vi "ERDFind.vi"(8 "error in":errorcluster, 10 "Read ERD List":T1[](array[typedef]) {"ERD Number" format="%.0x"}, 11 "ERD Data In":cluster{"ERD Number":u16, "Data":string}[](array[cluster])) -> (0 "error out":errorcluster, 1 "Read ERD List Out":T1[](array[typedef]) {"ERD Number" format="%.0x"}, 2 "ERD Data Out":cluster{"ERD Number":u16, "Data":string}[](array[cluster]) {"ERD Number" format="%.0x"}, 3 "ERD's No Found":string[](array[string]))   [LabVIEW 2021]
uses:
  Common/LabVIEW GEA2 Toolkit/GEA3/type defs/ERD Read Data In.ctl
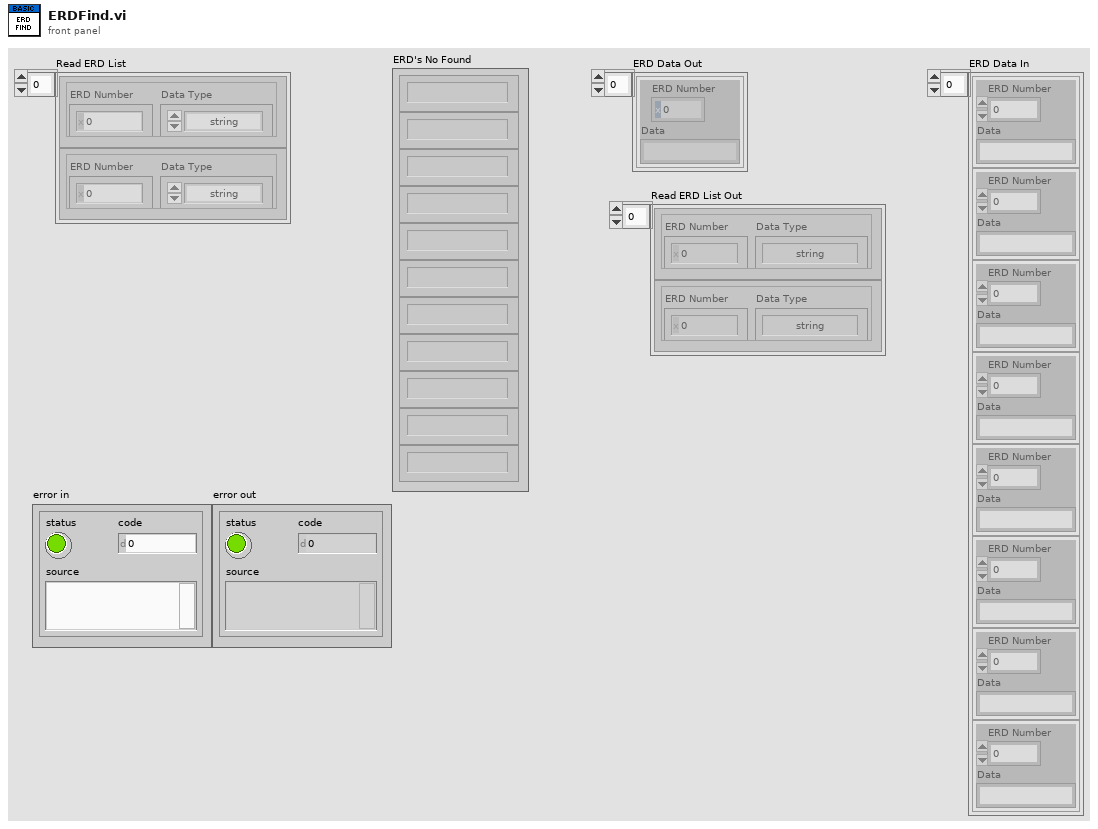
[diagram p1: front panel]
types:
  T1 = typedef "ERD Read Data In.ctl" = cluster{"ERD Number":u16, "Data Type":enum16{"string", "boolean", "uint8_t", "uint16_t", "uint32_t", "uint64_t", "int8_t", "int16_t", "int32_t", "int64_t"}}
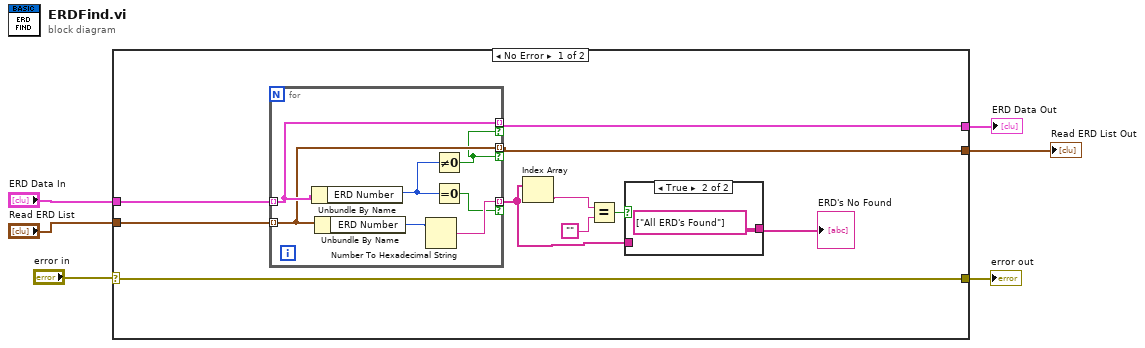
[diagram p0: block diagram]
diagram:
  n1 = case shown="No Error" "error in" {
    selector: "error in" -> [w11 w28]
    tunnel: [w11 w28] -> w5
    tunnel: [w10 w26] -> w3
    tunnel: [w9 w27] -> w4
    tunnel: "Read ERD List" -> [w8 w26]
    tunnel: "ERD Data In" -> [w7 w27]
    frame No Error {
      n2 = for {
        tunnel: w7 -> [w23] mode=indexing
        tunnel: w8 -> [w22] mode=indexing
        tunnel: [w24] -> w12 mode=indexing if=w21
        tunnel: [w23] -> w9 mode=indexing if=w20
        tunnel: [w22] -> w10 mode=indexing if=w20
        n3 = Unbundle By Name(w23) -> ("ERD Number"=w19:u16)
        n4 = Unbundle By Name(w22) -> ("ERD Number"=w25:u16)
        n5 = Number To Hexadecimal String(2:w25) -> (0:w24:string)  [unwired: 1 in]
        n6 = Not Equal To 0?(x=w19) -> (x != 0?=w20:bool)
        n7 = Equal To 0?(x=w19) -> (x = 0?=w21:bool)
      }
      n8 = Index Array(array=w12) -> (element=w14:string)  [unwired: 1 in]
      n9 = Equal?(x=w14, y="") -> (x = y?=w16:bool)
      n10 = case shown="True" w16 {
        tunnel: [w17 string[] ["All ERD's Found"]] -> w13
        tunnel: w12 -> [w17 _]
        frame False {
        }
        frame True {
        }
      }
      "ERD's No Found" <- w13
    }
    frame Error {
    }
  }
  "error out" <- w5
  "ERD Data Out" <- w4
  "Read ERD List Out" <- w3
